vi "Determine Warnings 3.vi"() -> ()   [LabVIEW 2014]
doc: "This VI will determine whether a temperature warning is needed based on the current, minimum, and maximum temperatures being inputted. \nInputs: Current Temp, Max Temp, Min Temp\nOutputs: Warning Text, Warning?\nEmma Gordon\n9/8/16"
panel:
  out "Warning?":bool
  out "Warning Text":string
  in  "Min Temp":dbl
  in  "Max Temp":dbl
  in  "Current Temp":dbl
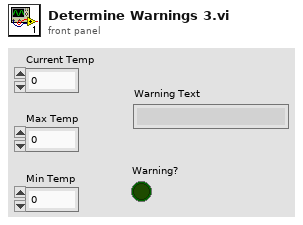
[diagram p1: front panel]
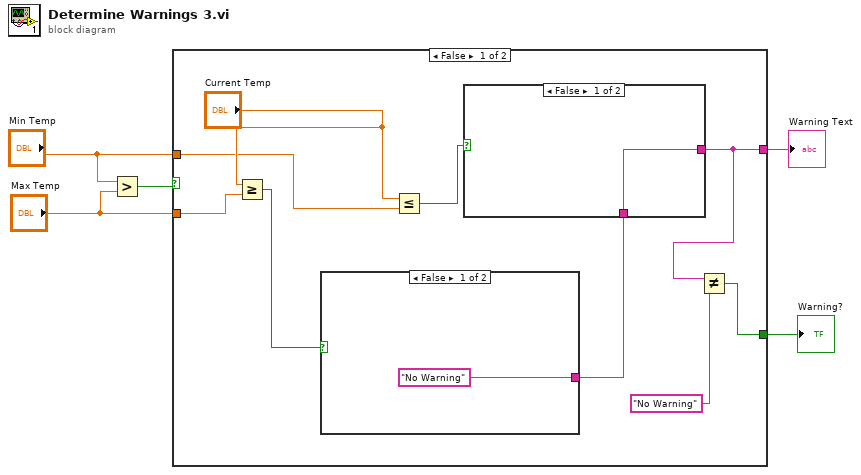
[diagram p0: block diagram]
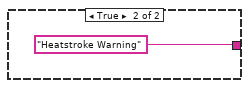
[diagram p2: hidden frame]
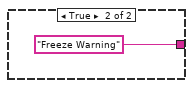
[diagram p3: hidden frame]
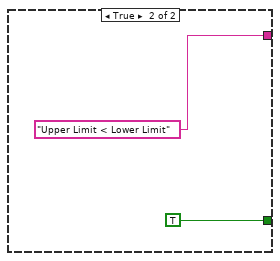
[diagram p4: hidden frame]
diagram:
  n1 = Greater?(x="Min Temp", y="Max Temp") -> (0:w1:bool)
  n2 = case shown="False" w1 {
    tunnel: [w10 "Upper Limit < Lower Limit"] -> w5
    tunnel: [w13 TRUE] -> w4
    tunnel: "Min Temp" -> [w12 _]
    tunnel: "Max Temp" -> [w11 _]
    frame False {
      n3 = Greater Or Equal?(x="Current Temp", y=w11) -> (x >= y?=w8:bool)
      n4 = case shown="False" w8 {
        tunnel: ["No Warning" "Heatstroke Warning"] -> w7
        frame False {
        }
        frame True {
        }
      }
      n5 = Less Or Equal?(x="Current Temp", y=w12) -> (x <= y?=w9:bool)
      n6 = case shown="False" w9 {
        tunnel: [w17 "Freeze Warning"] -> w10
        tunnel: w7 -> [w17 _]
        frame False {
        }
        frame True {
        }
      }
      n7 = Not Equal?(x=w10, y="No Warning") -> (x != y?=w13:bool)
    }
    frame True {
    }
  }
  "Warning Text" <- w5
  "Warning?" <- w4
